vi "Calibration Code for Sonar.vi"() -> ()   [LabVIEW 2014]
uses:
  <vilib>/Instr/_visa.llb/VISA Flush IO Buffer Mask.ctl
  <vilib>/Instr/_visa.llb/VISA Configure Serial Port (Instr).vi
  <vilib>/Utility/file.llb/Read From Spreadsheet File (DBL).vi
panel:
  in  "file path (dialog if empty)":path
  out "Waveform Graph":dbl[](graph)
  out "error out 2":errorcluster
  in  "Motor Direction":bool
  in  "?":bool
  out "Stop Engaged":bool
  out "Blinky Light":bool
  out "Sensor Head Position":dbl
  out "?":dbl(knob) scale=-800.0..800.0
  out "read buffer 2":string
  out "return count 2":u32
  out "Distance, in 2":dbl
  out "Waveform Chart 3":dbl(graph)
  in  "stop":bool
  out "IR Distance Reading":dbl
  out "Find starting position?":bool
  in  "VISA resource name 2":refnum<visa-resource-name>="COM3"
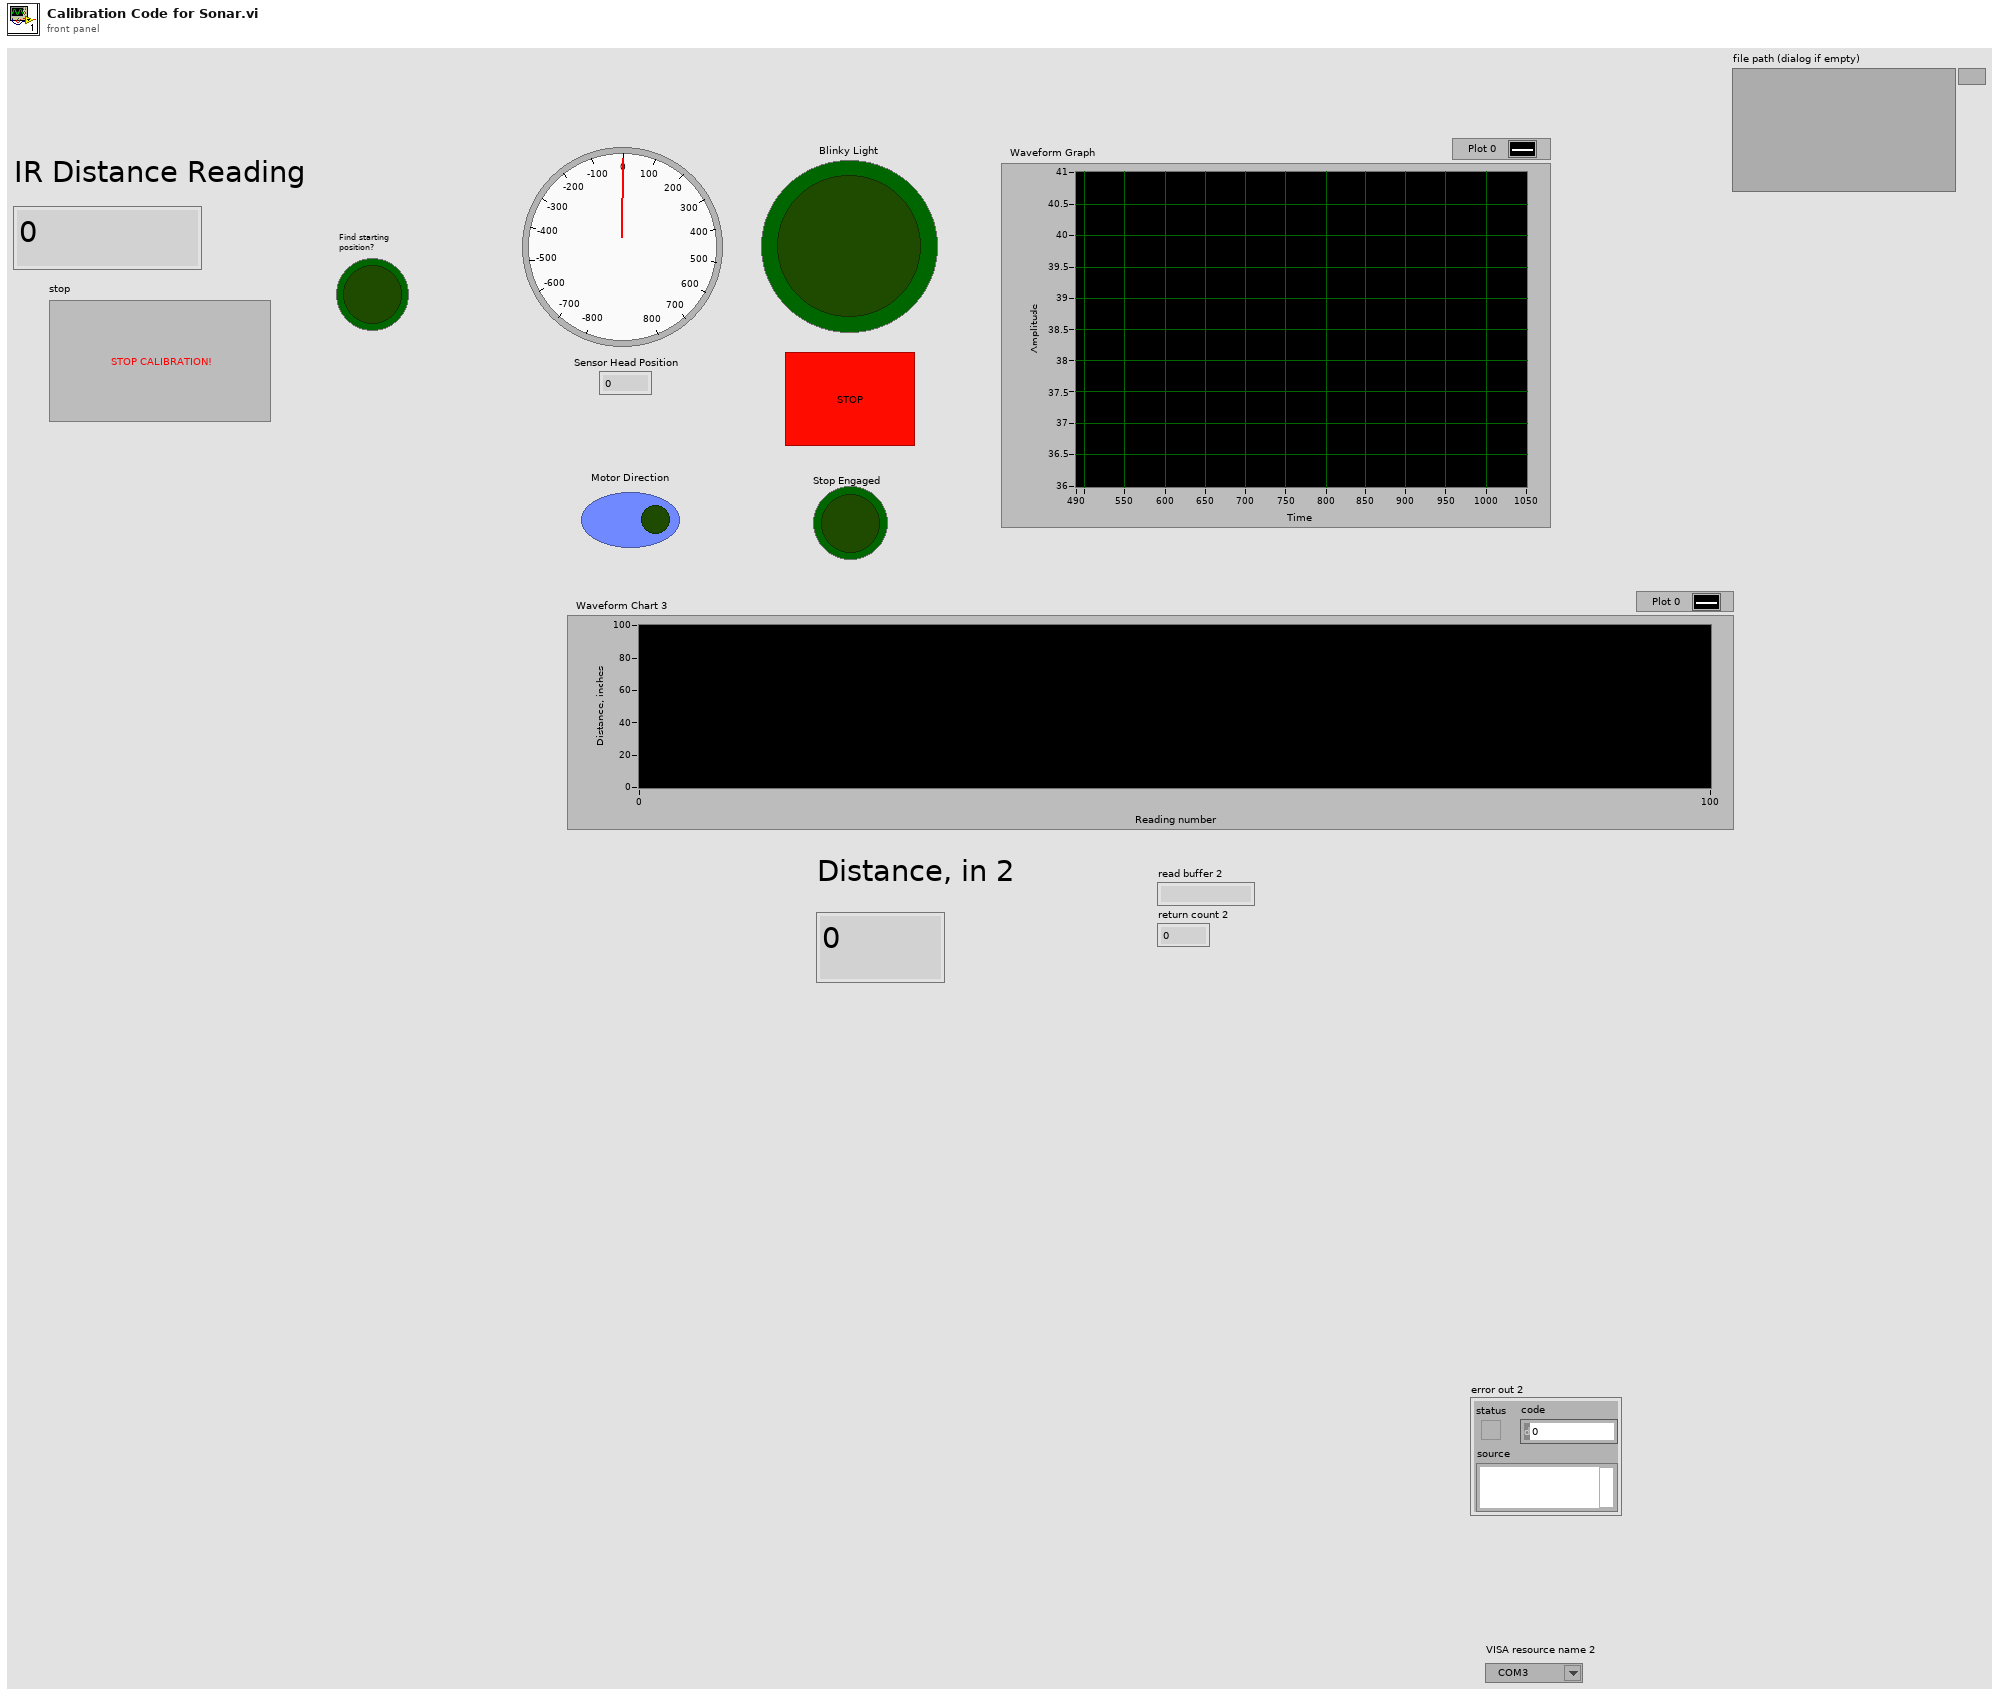
[diagram p1: front panel]
types:
  T1 = typedef "VISA Flush IO Buffer Mask.ctl" = u16
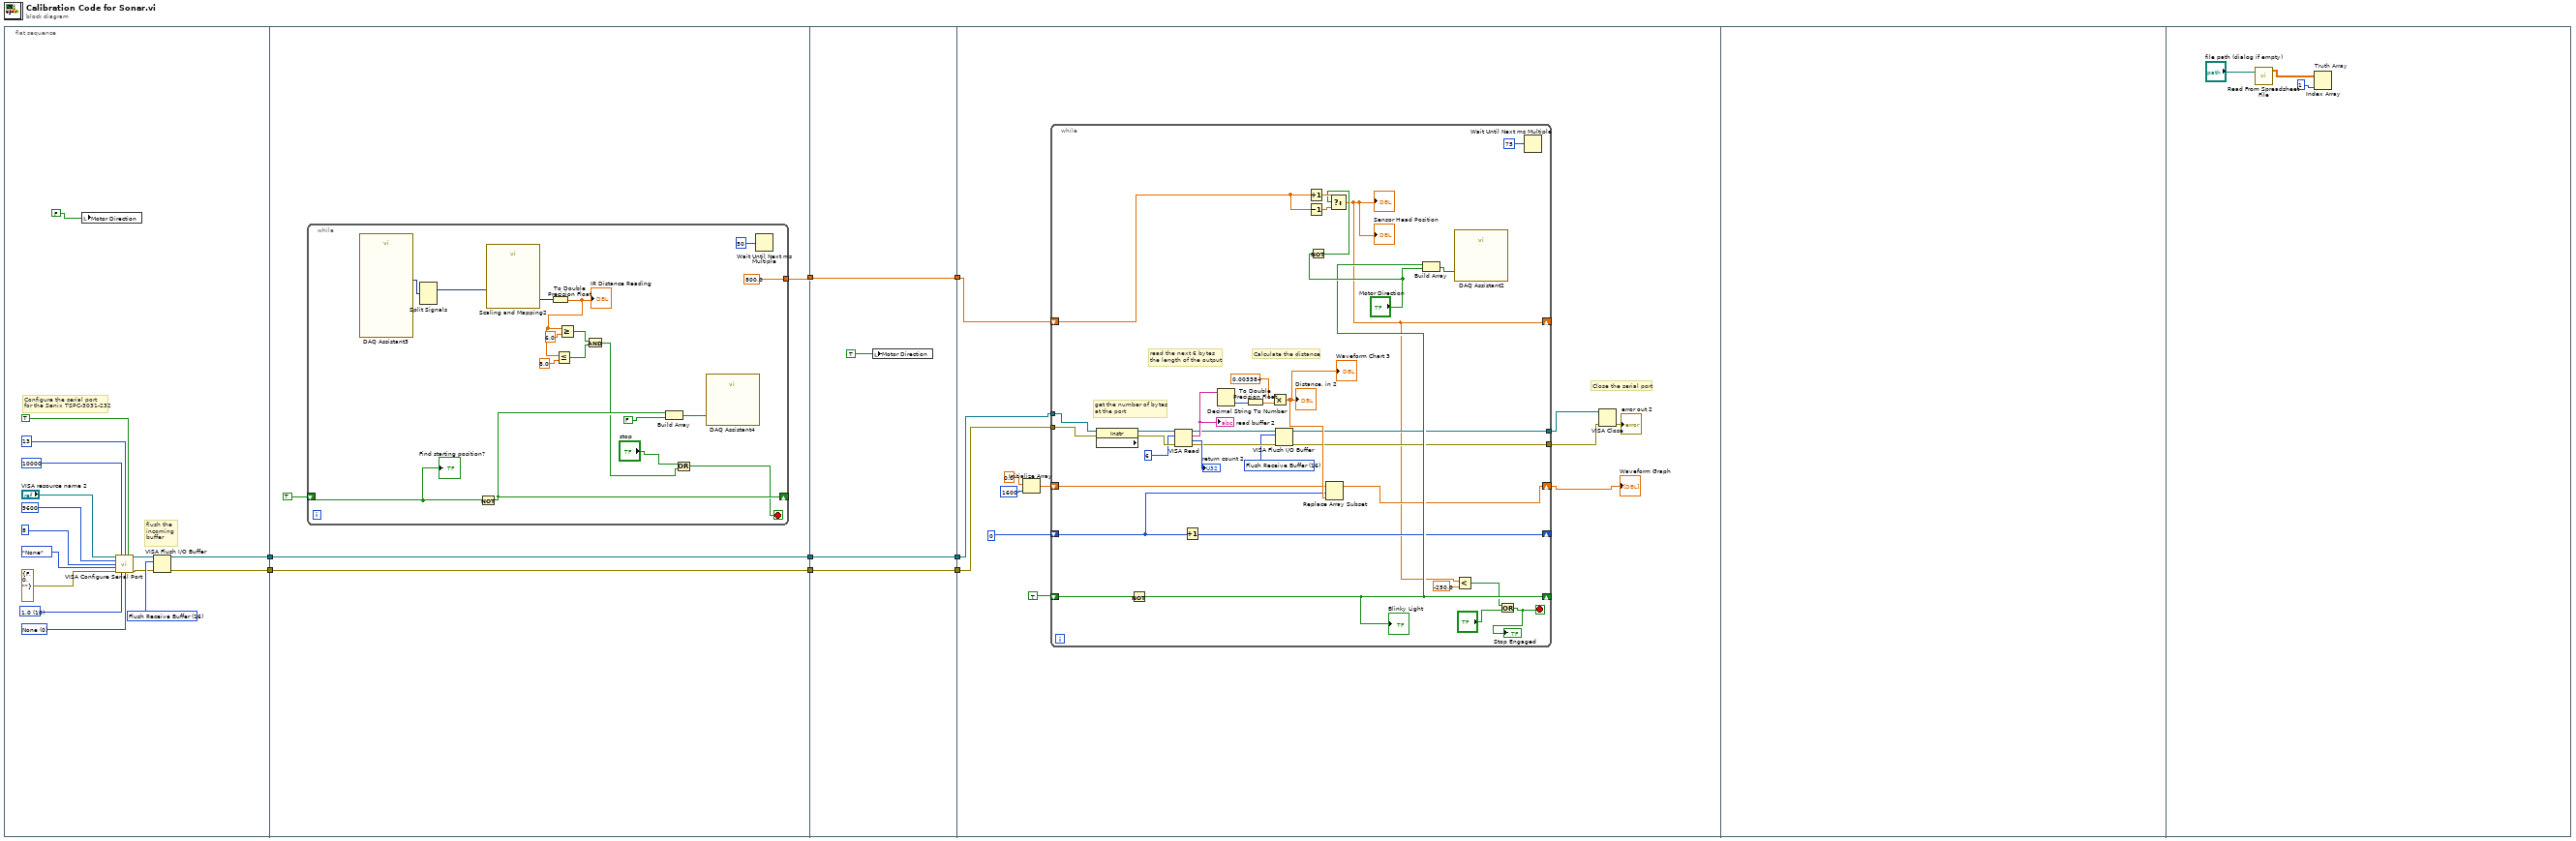
[diagram p0: block diagram]
diagram:
  n1 = flat-sequence {
    tunnel: [w11] -> w8
    tunnel: [w10] -> w7
    tunnel: w8 -> [w28]
    tunnel: w7 -> [w27]
    tunnel: [w25] -> w6
    tunnel: [w28] -> w5
    tunnel: [w27] -> w4
    tunnel: w6 -> [w49]
    tunnel: w5 -> [w48]
    tunnel: w4 -> [w47]
    tunnel: [w49] -> w3
    tunnel: [w48] -> w2
    tunnel: [w47] -> w1
    tunnel: w3 -> [w55]
    tunnel: w2 -> [w54]
    tunnel: w1 -> [w53]
    frame #0 {
      w14 = T1 16 items=["Flush Receive Buffer"=16, "Write Transmit Buffer to Device"=32, "Flush Receive Buffer (No I/O)"=64, "Flush Transmit Buffer"=128] ("Mask")
      w18 = u16 0 items=["None", "XON/XOFF", "RTS/CTS", "XON/XOFF & RTS/CTS", "DTR/DSR", "XON/XOFF & DTR/DSR"] ("flow control (0:none)")
      w20 = u16 10 items=["1.0"=10, "1.5"=15, "2.0"=20] ("stop bits (10: 1 bit)")
      # "flush the \nincoming \nbuffer"
      # "Configure the serial port\nfor the Senix TSPC-3031-232"
      n2 = local write "Motor Direction"(FALSE) -> ()
      n3 = call-poly "VISA Configure Serial Port"("VISA resource name"="VISA resource name 2", "timeout (10sec)"=u32 10000, "termination char\n(0xA = '\\n' = LF)"=u8 13 ("termination char\n(0xA = '\\n' = LF)"), "Enable Termination\nChar (T)"=TRUE ("Enable Termination\nChar (T)"), "baud rate (9600)"=u32 9600, "data bits (8)"=u16 8, "parity (0:none)"=enum16{"None", "Odd", "Even", "Mark", "Space"}."None", "error in (no error)"=errorcluster {"status"=FALSE, "code"=0, "source"=""}, "stop bits (10: 1 bit)"=w20, "flow control (0:none)"=w18) -> ("VISA resource name out"=w13:refnum<visa-resource-name>, "error out"=w12:errorcluster)  [unwired: 4 in]
      n4 = VISA Flush I/O Buffer(VISA resource name=w13, mask (16)=w14, error in (no error)=w12) -> (VISA resource name out=w11:refnum<visa-resource-name>, error out=w10:errorcluster)
    }
    frame #1 {
      n5 = while {
        tunnel: [800.0] -> w25
        shift-right: [w44] -> _
        shift-left: TRUE -> [w42]
        stop <- w31 stop-if-true
        n6 = call "DAQ Assistant3"() -> ("data"=w40:dynamicdata)  [unwired: 16 in, 3 out]
        n7 = Split Signals "Split Signals"(w40) -> (w41:dynamicdata)  [unwired: 5 in, 4 out]
        n8 = Not(x=w42) -> (.not. x?=w44:bool)
        n9 = call "Scaling and Mapping2"("Signals"=w41) -> ("Scaled Signals"=w35:dynamicdata)  [unwired: 9 in, 1 out]
        n10 = To Double Precision Float(number=w35) -> (double precision float=w34:dbl)
        "IR Distance Reading" <- w34
        n11 = Less Or Equal?(x=w34, y=8.0) -> (x <= y?=w36:bool)
        n12 = Greater Or Equal?(x=w34, y=6.0) -> (x >= y?=w37:bool)
        n13 = And(x=w37, y=w36) -> (x .and. y?=w32:bool)
        n14 = Build Array(w44, FALSE) -> (w45:bool[])
        n15 = Or(x="stop", y=w32) -> (x .or. y?=w31:bool)
        n16 = call "DAQ Assistant4"("data"=w45) -> ()  [unwired: 17 in, 2 out]
        n17 = Wait Until Next ms Multiple(millisecond multiple=50) -> ()  [unwired: 1 out]
        "Find starting position?" <- w42
      }
    }
    frame #2 {
      n18 = local write "Motor Direction"(TRUE) -> ()
    }
    frame #3 {
      # "Close the serial port"
      n19 = Initialize Array(0.0 ("element"), 1600 ("dimension size")) -> (w60:dbl[])
      n20 = while {
        shift-right: [w62] -> _
        shift-left: w55 -> [w92]
        shift-right: [w73] -> _
        shift-left: TRUE -> [w87]
        tunnel: w54 -> [w72]
        tunnel: w53 -> [w71]
        shift-right: [w68] -> w56
        shift-left: w60 -> [w70]
        shift-right: [w67] -> _
        shift-left: 0 ("dimension size") -> [w69]
        tunnel: [w66] -> w58
        tunnel: [w65] -> w57
        stop <- w86 stop-if-true
        w76 = T1 16 items=["Flush Receive Buffer"=16, "Write Transmit Buffer to Device"=32, "Flush Receive Buffer (No I/O)"=64, "Flush Transmit Buffer"=128] ("Mask")
        # "Calculate the distance"
        # "read the next 6 bytes\nthe length of the output"
        # "get the number of bytes\nat the port"
        n21 = property class="Instr" props=["Serial Settings:Number of Bytes at Serial Port"](reference=w72, error in=w71) -> (reference out=w85:refnum<visa-resource-name>, error out=w84:errorcluster)  [unwired: 1 out]
        n22 = Not(x=w87) -> (.not. x?=w73:bool)
        "Blinky Light" <- w73
        n23 = VISA Read(VISA resource name=w85, byte count=u32 6, error in (no error)=w84) -> (VISA resource name out=w78:refnum<visa-resource-name>, read buffer=w82:string, return count=→"return count 2":u32, error out=w77:errorcluster)
        "read buffer 2" <- w82
        n24 = Increment(x=w69) -> (x+1=w67:i32)
        n25 = Decimal String To Number(string=w82) -> (number=w81:i32)  [unwired: 2 in, 1 out]
        n26 = To Double Precision Float(number=w81) -> (double precision float=w80:dbl)
        n27 = Multiply(x=0.003384, y=w80) -> (x*y=w74:dbl)
        "Distance, in 2" <- w74
        "Waveform Chart 3" <- w74
        n28 = VISA Flush I/O Buffer(VISA resource name=w78, mask (16)=w76, error in (no error)=w77) -> (VISA resource name out=w66:refnum<visa-resource-name>, error out=w65:errorcluster)
        n29 = Increment(x=w92) -> (x+1=w94:dbl)
        n30 = Decrement(x=w92) -> (x-1=w93:dbl)
        n31 = Not(x="Motor Direction") -> (.not. x?=w90:bool)
        n32 = Replace Array Subset(array=w70, new element=w74, index=w69) -> (w68:dbl[])
        n33 = Select(t=w94, s=w90, f=w93) -> (s? t:f=w62:dbl)
        "Sensor Head Position" <- w62
        "?" <- w62
        n34 = Build Array(w73, "Motor Direction") -> (w88:bool[])
        n35 = call "DAQ Assistant2"("data"=w88) -> ()  [unwired: 17 in, 2 out]
        n36 = Less?(x=w62, y=-250.0) -> (x < y?=w64:bool)
        n37 = Or(x=w64, y="?") -> (x .or. y?=w86:bool)
        "Stop Engaged" <- w86
        n38 = Wait Until Next ms Multiple(millisecond multiple=75) -> ()  [unwired: 1 out]
      }
      "Waveform Graph" <- w56
      n39 = VISA Close(VISA resource name=w58, error in (no error)=w57) -> (error out=→"error out 2":errorcluster)
    }
    frame #4 {
    }
    frame #5 {
      n40 = call-poly <vilib>:"Read From Spreadsheet File.vi"("file path (dialog if empty)"="file path (dialog if empty)") -> ("all rows"=w97:dbl[][])  [unwired: 6 in, 4 out]
      n41 = Index Array "Truth Array"(array=w97, index (col)=1 ("index")) -> ()  [unwired: 1 in, 1 out]
    }
  }
